vi "Q Vision_Object Params Global.vi"(7 "Action":enum16{"Get", "Set"}(ring), 8 "error in (no error)":errorcluster, 11 "Object Params in":T1) -> (0 "error out":errorcluster, 3 "Object Params out":T1)   [LabVIEW 2016]
uses:
  Typedefs/typedef_cluster_Object Params.ctl
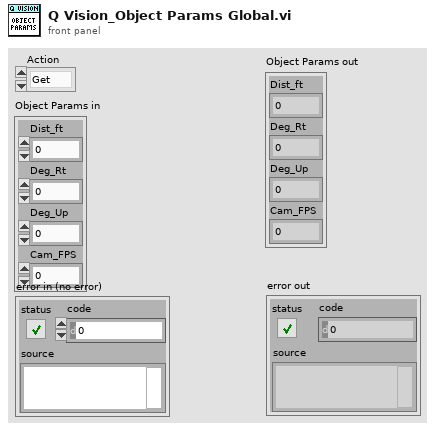
[diagram p1: front panel]
types:
  T1 = typedef "typedef_cluster_Object Params.ctl" = cluster{"Dist_ft":dbl, "Deg_Rt":dbl, "Deg_Up":dbl, "Cam_FPS":dbl}
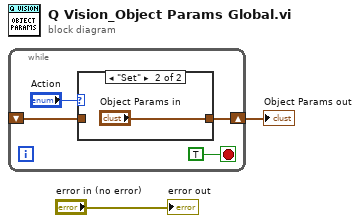
[diagram p0: block diagram]
diagram:
  n1 = while {
    shift-right: [w5] -> w2
    shift-left: _ -> [w4]
    stop <- TRUE stop-if-true
    n2 = case shown="\"Set\"" "Action" {
      tunnel: [w7 "Object Params in"] -> w5
      tunnel: w4 -> [w7 _]
      frame "Get", Default {
      }
      frame "Set" {
      }
    }
  }
  "Object Params out" <- w2
  "error out" <- "error in (no error)"
